vi "Handle Error.vi"(8 "error in (no error)":errorcluster, 11 "LocalReport in":refnum<class "LocalReport.lvclass">) -> (0 "error out":errorcluster, 2 "stop actor?":bool=TRUE, 3 "LocalReport out":refnum<class "LocalReport.lvclass">)   [LabVIEW 2019, in "LocalReport.lvlib" / "LocalReport.lvclass"]
doc: "(<B>Filename</B>: Actor Framework.lvlib:Actor.lvclass:Handle Error.vi)\n\nDefines how the actor handles an error that occurred while processing a message. By default, this method does nothing except stop the actor."
uses:
  LocalReport.lvclass
  <vilib>/NI/Event Source Actor/Event Source/Event Source/Event Source.lvclass
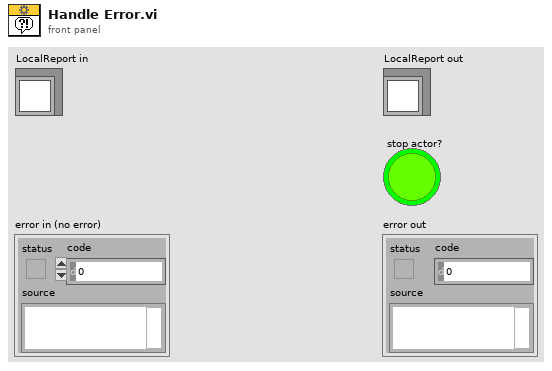
[diagram p1: front panel]
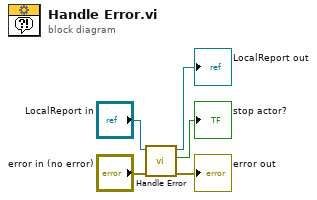
[diagram p0: block diagram]
diagram:
  n1 = call-parent "Handle Error.vi"("error in (no error)"="error in (no error)", "Actor in"="LocalReport in") -> ("error out"=→"error out":errorcluster, "stop actor?"=→"stop actor?":bool, "Actor out"=→"LocalReport out":refnum<class "LocalReport.lvclass">)  [unwired: 7 in]
